vi "耐久性测试输出调用01.vi"(0 "电流":dbl, 5 "时长":dbl, 9 "字符串":string, 11 "输出簇":cluster{"电压1":refnum<vi>, "电流1":refnum<vi>}) -> ()   [LabVIEW 2020]
uses:
  <vilib>/Utility/miscctls.llb/LVDateTimeRec.ctl
panel:
  out "输出 3":dbl
  out "输出 2":dbl
  out "路径":path
  out "错误输出":errorcluster
  out "元素":string
  out "数值 3":i32
  out "Numeric":i32
  in  "数值":u32
  out "输出 1":dbl
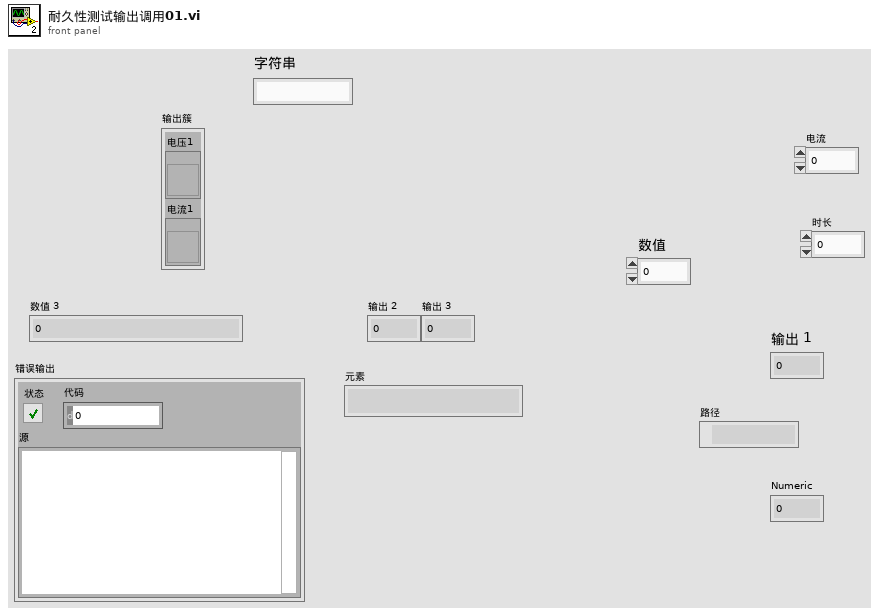
[diagram p1: front panel]
types:
  T1 = enum16{"open", "replace", "create", "open or create", "replace or create", "replace or create with confirmation"}
  T2 = typedef "LVDateTimeRec.ctl" = cluster{"fractional second":dbl, "second":i32, "minute":i32, "hour":i32, "day of month":i32, "month":i32, "year":i32, "day of week":i32, "day of year":i32, "DST":i32}
  T3 = enum16{"open", "open or create", "create or replace", "create", "open (read-only)"}
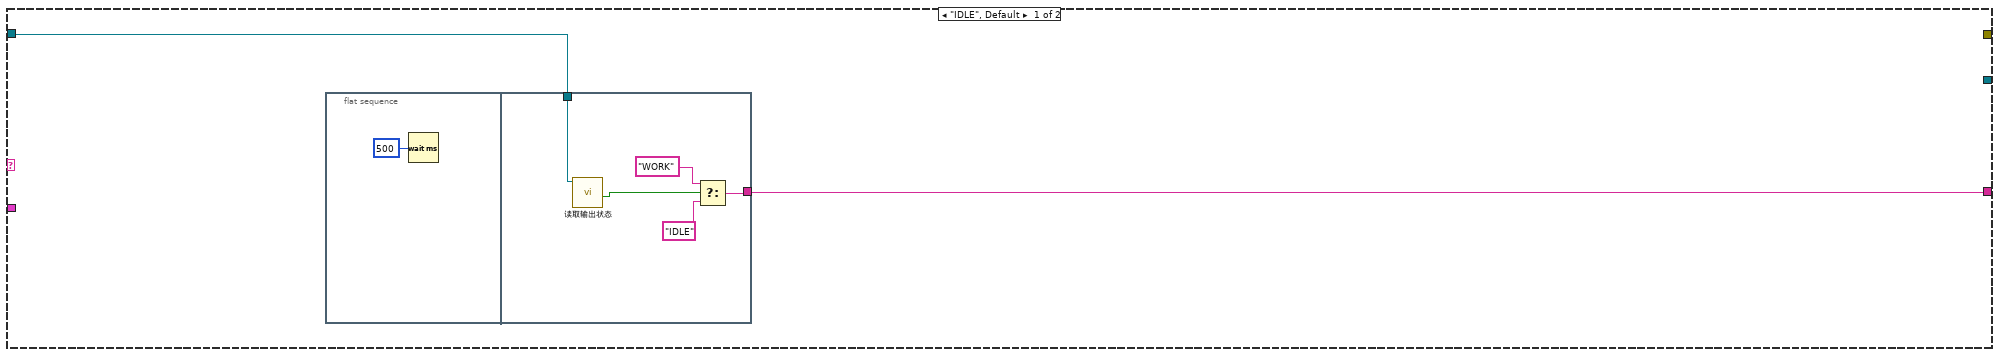
[diagram p2: hidden frame]
diagram:
  n1 = Current VI's Path() -> (path=w5:path)
  n2 = Strip Path(path=w5) -> (stripped path=w6:path)  [unwired: 1 out]
  n3 = Strip Path(path=w6) -> (stripped path=w7:path)  [unwired: 1 out]
  n4 = Path To String(path=w7) -> (string=w8:string)
  n5 = flat-sequence {
    tunnel: ["字符串"] -> w26
    tunnel: [w36] -> w27
    tunnel: w26 -> [w36]
    tunnel: [w44] -> w33
    tunnel: [w43] -> w32
    tunnel: [w42] -> w28
    tunnel: w27 -> [w41]
    tunnel: w33 -> [w54]
    tunnel: w32 -> [w53]
    tunnel: [w46] -> w31
    tunnel: [w45] -> w30
    tunnel: w31 -> [w93]
    tunnel: w30 -> [w92]
    tunnel: [w91] -> w29
    tunnel: [w90] -> w20
    tunnel: w29 -> [w121]
    tunnel: w20 -> [w119]
    frame #0 {
      n6 = property on="数值" class="DigNum (严格)"("Value"=i64 0 ("数值")) -> ()  [unwired: 2 in, 2 out]
    }
    frame #1 {
      n7 = VISA Close(VISA resource name="字符串") -> ()  [unwired: 1 in, 1 out]
    }
    frame #2 {
    }
    frame #3 {
      n8 = VISA Open(VISA resource name=w41) -> (VISA resource name=w42:refnum<visa-resource-name>, error out=w39:errorcluster)  [unwired: 4 in]
      n9 = call "remote.vi"("error in (no error)"=w39, "VISA resource name"=w42) -> ("error out"=w37:errorcluster, "VISA resource name out"=w38:refnum<visa-resource-name>)  [unwired: 8 in]
      n10 = call "enableoutput.vi"("error in (no error)"=w37, "Enable OutPut(True)"=FALSE, "VISA resource name"=w38) -> ("error out"=w43:errorcluster, "VISA resource name out"=w44:refnum<visa-resource-name>)  [unwired: 7 in]
    }
    frame #4 {
      n11 = flat-sequence {
        tunnel: w54 -> [w59]
        tunnel: w53 -> [w58]
        tunnel: [w56] -> w52
        tunnel: [w55] -> w51
        tunnel: w52 -> [w65]
        tunnel: w51 -> [w64]
        tunnel: [w61] -> w50
        tunnel: [w60] -> w49
        tunnel: w50 -> [w71]
        tunnel: w49 -> [w70]
        tunnel: [w68] -> w48
        tunnel: [w67] -> w47
        tunnel: w48 -> [w77]
        tunnel: w47 -> [w76]
        tunnel: [w73] -> w46
        tunnel: [w72] -> w45
        frame #0 {
          n12 = call "priority.vi"("error in (no error)"=w58, "字符串"="CURR", "VISA resource name"=w59) -> ("error out"=w55:errorcluster, "VISA resource name out"=w56:refnum<visa-resource-name>)  [unwired: 7 in]
        }
        frame #1 {
          n13 = call "初始化电压电流.vi"("error in (no error)"=w64, "输入 2"=0.1, "输入 1"=15.0, "VISA resource name"=w65) -> ("error out"=w60:errorcluster, "VISA resource name out"=w61:refnum<visa-resource-name>)  [unwired: 6 in]
        }
        frame #2 {
          n14 = call "限制电流.vi"("error in (no error)"=w70, "OCP Delay(0)"=3.0, "数值"=120.0 ("OCP Level(0)"), "VISA resource name"=w71) -> ("error out"=w67:errorcluster, "VISA resource name out"=w68:refnum<visa-resource-name>)  [unwired: 6 in]
        }
        frame #3 {
          n15 = call "限制电压.vi"("error in (no error)"=w76, "OVP Delay(0)"=3.0, "OVP Level(0)"=20.0, "VISA resource name"=w77) -> ("error out"=w72:errorcluster, "VISA resource name out"=w73:refnum<visa-resource-name>)  [unwired: 6 in]
        }
      }
    }
    frame #5 {
      n16 = flat-sequence {
        tunnel: w93 -> [w98]
        tunnel: w92 -> [w97]
        tunnel: [w96] -> w89
        tunnel: [w95] -> w88
        tunnel: "电流" -> [w94]
        tunnel: w89 -> [w101]
        tunnel: w88 -> [w102]
        tunnel: [w100] -> w87
        tunnel: [w99] -> w86
        tunnel: w80 -> [w112]
        tunnel: w87 -> [w111]
        tunnel: [w111] -> w85
        tunnel: [w110] -> w84
        tunnel: w86 -> [w110]
        tunnel: w85 -> [w114]
        tunnel: [w114] -> w83
        tunnel: w84 -> [w113]
        tunnel: [w113] -> w82
        tunnel: [w117] -> w91
        tunnel: w83 -> [w118]
        tunnel: w82 -> [w116]
        tunnel: [w115] -> w90
        frame #0 {
          n17 = call "设置电流.vi"("error in (no error)"=w97, "输入 1"=w94, "VISA resource name"=w98) -> ("error out"=w95:errorcluster, "VISA resource name out"=w96:refnum<visa-resource-name>)  [unwired: 7 in]
        }
        frame #1 {
          n18 = First Call?() -> (First Call?: T/F=w103:bool)
          n19 = case shown="真" w103 {
            tunnel: w101 -> [w104 w109]
            tunnel: w102 -> [_ w108]
            tunnel: [w104 w106] -> w100
            tunnel: [_ w105] -> w99
            frame False {
            }
            frame True {
              n20 = call "enableoutput.vi"("error in (no error)"=w108, "Enable OutPut(True)"=TRUE, "VISA resource name"=w109) -> ("error out"=w105:errorcluster, "VISA resource name out"=w106:refnum<visa-resource-name>)  [unwired: 7 in]
            }
          }
        }
        frame #2 {
          n21 = Wait (ms)(milliseconds to wait=w112) -> ()  [unwired: 1 out]
        }
        frame #3 {
        }
        frame #4 {
          n22 = call "remote.vi"("error in (no error)"=w116, "VISA resource name"=w118) -> ("error out"=w115:errorcluster, "VISA resource name out"=w117:refnum<visa-resource-name>)  [unwired: 8 in]
        }
      }
      n23 = Multiply(x="时长", y=3600000.0) -> (x*y=w80:dbl)
      "输出 1" <- "电流"
    }
    frame #6 {
      n24 = flat-sequence {
        tunnel: w121 -> [w125]
        tunnel: [w124] -> w120
        tunnel: w119 -> [w122]
        tunnel: w120 -> [w126]
        frame #0 {
          n25 = call "enableoutput.vi"("error in (no error)"=w122, "Enable OutPut(True)"=FALSE, "VISA resource name"=w125) -> ("VISA resource name out"=w124:refnum<visa-resource-name>)  [unwired: 7 in, 1 out]
        }
        frame #1 {
          n26 = VISA Close(VISA resource name=w126) -> ()  [unwired: 1 in, 1 out]
        }
        frame #2 {
          n27 = flat-sequence {
            tunnel: [w140] -> w132
            tunnel: [w139] -> w131
            tunnel: [w138] -> w130
            tunnel: w132 -> [w164]
            tunnel: w131 -> [w165]
            tunnel: [w164] -> w127
            tunnel: [w165] -> w128
            tunnel: w130 -> [w163]
            tunnel: [w163] -> w129
            tunnel: w129 -> [w188]
            tunnel: w128 -> [w192]
            tunnel: w127 -> [w191]
            frame #0 {
              n28 = property on="路径" class="Path"() -> ("Value"=w137:path)  [unwired: 2 in, 2 out]
              n29 = Open/Create/Replace File(file path (use dialog)=w137, operation (0:open)=T1."open" ("操作(0:open)")) -> (refnum out=w142:refnum<file>, error out=w141:errorcluster)  [unwired: 4 in, 1 out]
              n30 = Read from Text File(file (use dialog)=w142, count=-1 ("计数"), error in=w141) -> (refnum out=w135:refnum<file>, text=w136:string[], error out=w133:errorcluster)  [unwired: 1 in, 1 out]
              n31 = for {
                tunnel: [w148] -> w140 mode=indexing
                tunnel: [w147] -> w139 mode=indexing
                tunnel: [w151] -> w138 mode=indexing
                tunnel: w136 -> [w144] mode=indexing
                i -> [w146]
                n32 = Search/Split String(string=w144, search string/char (-)="电流：" ("正则表达式")) -> (substring before match=w159:string, match + rest of string=w150:string)  [unwired: 1 in, 1 out]
                n33 = Scan From String(format string="%d-%d-%d %d:%d:%d" ("格式字符串"), input string=w159) -> (output 1=w158:i32, output 2=w157:i32, output 3=w156:i32, output 4=w155:i32, output 5=w154:i32, output 6=w153:i32)  [unwired: 8 in, 3 out]
                n34 = Bundle By Name(cluster=T2 {"fractional second"=0.9035696983337402, "second"=34, "minute"=35, "hour"=15, "day of month"=21, "month"=2, "year"=2022, "day of week"=2, "day of year"=52, "DST"=0} ("日期时间记录"), "second"=w153, "minute"=w154, "hour"=w155, "day of month"=w156, "month"=w157, "year"=w158) -> (w152:T2)
                n35 = Scan From String(format string="电流：%f 电压：%f" ("格式字符串"), input string=w150) -> (error out=w145:errorcluster, output 1=w148:dbl, output 2=w147:dbl)  [unwired: 4 in, 2 out]
                n36 = call <vilib>:"Clear Errors.vi"("error in (no error)"=w145) -> ()  [unwired: 5 in, 2 out]
                n37 = Date/Time To Seconds(2:w152) -> (0:w151:timestamp)  [unwired: 1 in]
                "元素" <- w144
                "数值 3" <- w146
              }
              n38 = Close File(refnum=w135, error in=w133) -> ()  [unwired: 2 out]
            }
            frame #1 {
            }
            frame #2 {
              w182 = "数据" ("组名称")
              n39 = Array Size(array=w188) -> (size(s)=w187:i32)
              n40 = Array Max & Min(array=w192) -> (max value=w205:dbl, max index (indices)=w200:i32, min value=w204:dbl, min index (indices)=w199:i32)
              n41 = Array Max & Min(array=w191) -> (max value=w207:dbl, max index (indices)=w201:i32, min value=w208:dbl, min index (indices)=w202:i32)
              n42 = Index Array(array=w188, index=0 ("索引")) -> (element=w185:timestamp)
              n43 = Decrement(x=w187) -> (x-1=w186:i32)
              n44 = Build Array(w204, w205, w200, w199) -> (w203:dbl[])
              n45 = Build Array(w208, w207, w202, w201) -> (w206:dbl[])
              n46 = Index Array(array=w188, index=w186) -> (element=w184:timestamp)
              n47 = call <vilib>:"Application Directory.vi"() -> ("Application Directory"=w166:path)
              n48 = Path To String(path=w166) -> (string=w171:string)
              n49 = Get Date/Time In Seconds() -> (seconds since 1Jan1904=w224:timestamp)
              n50 = Format Date/Time String(time format string (%c)="%Y-%m-%d-%H-%M-%S" ("时间格式字符串(%c)"), seconds (now)=w224) -> (date/time string=w173:string)  [unwired: 1 in]
              n51 = Concatenate Strings(w171, "\\" ("字符串"), w173, ".tdms" ("字符串")) -> (w225:string)
              n52 = String To Path(string=w225) -> (path=w226:path)
              n53 = Build Array(w185, w184) -> (w183:timestamp[])
              n54 = TDMS Open(5:FALSE ("创建索引文件？(T)"), 10:T3."create or replace" ("操作(0:open)"), 11:w226) -> (0:w179:errorcluster, 3:w181:refnum<k34>)  [unwired: 4 in]
              n55 = Build Array("电解水实验" ("组名称"), "孙成，王彪" ("组名称"), w173, "极化曲线" ("组名称")) -> (w172:string[])
              n56 = TDMS Set Properties(5:w172, 7:string[] ["Title", "Author", "Date/Time", "type"] ("属性名称"), 8:w179, 11:w181) -> (0:w178:errorcluster, 3:w180:refnum<k34>)  [unwired: 2 in, 2 out]
              n57 = TDMS Set Properties(5:w183, 7:string[] ["最小值", "最大值"] ("属性名称"), 8:w178, 9:"测试时间" ("通道名称"), 10:w182, 11:w180) -> (0:w215:errorcluster, 3:w216:refnum<k34>)  [unwired: 2 out]
              n58 = TDMS Set Properties(5:w206, 7:string[] ["最小值", "最大值", "最小索引", "最大索引"] ("属性名称"), 8:w215, 9:"电流" ("通道名称"), 10:w182, 11:w216) -> (0:w209:errorcluster, 3:w212:refnum<k34>)  [unwired: 2 out]
              n59 = TDMS Set Properties(5:w203, 7:string[] ["最小值", "最大值", "最小索引", "最大索引"] ("属性名称"), 8:w209, 9:"电压" ("通道名称"), 10:w182, 11:w212) -> (0:w167:errorcluster, 3:w168:refnum<k34>)  [unwired: 2 out]
              n60 = TDMS Write(0:w168, 5:"数据" ("组名称输入（无标题）"), 7:string[] ["电流"] ("通道名输入（无标题）"), 9:w191, 11:w167) -> (4:w195:refnum<k34>, 15:w194:errorcluster)  [unwired: 1 in, 2 out]
              n61 = TDMS Write(0:w195, 5:"数据" ("组名称输入（无标题）"), 7:string[] ["电压"] ("通道名输入（无标题）"), 9:w192, 11:w194) -> (4:w170:refnum<k34>, 15:w169:errorcluster)  [unwired: 1 in, 2 out]
              n62 = TDMS Close(8:w169, 11:w170) -> (0:→"错误输出":errorcluster)  [unwired: 1 out]
            }
          }
        }
        frame #3 {
          n63 = Request Deallocation(TRUE ("标志")) -> ()
        }
        frame #4 {
          n64 = Stop(stop? (T)=TRUE ("停止？(T)")) -> ()
        }
      }
    }
  }
  n65 = Get Date/Time In Seconds() -> (seconds since 1Jan1904=w10:timestamp)
  n66 = Format Date/Time String(time format string (%c)="%y-%m-%d[%H-%M]", seconds (now)=w10) -> (date/time string=w13:string)  [unwired: 1 in]
  n67 = Concatenate Strings(w8, "\\" ("string"), "耐久性\\" ("string"), w13) -> (w3:string)
  n68 = String To Path(string=w3) -> (path=w4:path)
  n69 = Create Folder(path (use dialog)=w4) -> (created path=w2:path)  [unwired: 2 in, 2 out]
  n70 = Path To String(path=w2) -> (string=w17:string)
  n71 = Concatenate Strings(w17, "\\" ("string"), "数据.txt" ("string")) -> (w16:string)
  n72 = String To Path(string=w16) -> (path=w15:path)
  "路径" <- w15
  n73 = Open/Create/Replace File(file path (use dialog)=w15, operation (0:open)=T1."replace or create" ("操作(0:open)")) -> (refnum out=w14:refnum<file>, error out=w23:errorcluster)  [unwired: 4 in, 1 out]
  n74 = while {
    shift-right: [w232] -> _
    shift-left: "IDLE" -> [w238]
    tunnel: w28 -> [w237]
    tunnel: w14 -> [w236]
    tunnel: w23 -> [w235]
    tunnel: [w234] -> w22
    tunnel: [w233] -> w21
    tunnel: "输出簇" -> [w229]
    i -> [w231]
    stop <- FALSE stop-if-true
    n75 = Wait (ms)(milliseconds to wait=u32 500 ("等待时间（毫秒）")) -> ()  [unwired: 1 out]
    n76 = case shown="\"WORK\"" w238 {
      tunnel: [w241 w269] -> w232
      tunnel: w237 -> [w240 w277]
      tunnel: w236 -> [_ w276]
      tunnel: w235 -> [_ w274]
      tunnel: [_ w271] -> w234
      tunnel: [_ w270] -> w233
      tunnel: w229 -> [_ w250]
      frame "IDLE", Default {
        n77 = flat-sequence {
          tunnel: [w244] -> w241
          tunnel: w240 -> [w243]
          frame #0 {
            n78 = Wait (ms)(milliseconds to wait=u32 500 ("等待时间（毫秒）")) -> ()  [unwired: 1 out]
          }
          frame #1 {
            n79 = call "读取输出状态.vi"("VISA resource name"=w243) -> ("x = y?"=w247:bool)  [unwired: 7 in, 3 out]
            n80 = Select(t="WORK", s=w247, f="IDLE") -> (s? t:f=w244:string)
          }
        }
      }
      frame "WORK" {
        n81 = Unbundle By Name(w250) -> ("电压1"=w248:refnum<vi>, "电流1"=w249:refnum<vi>)
        n82 = flat-sequence {
          tunnel: [w286] -> w280
          tunnel: [w285] -> w279
          tunnel: w277 -> [w284]
          tunnel: w276 -> [w282]
          tunnel: [w283] -> w275
          tunnel: w274 -> [w283]
          tunnel: [w282] -> w273
          tunnel: [w281] -> w272
          tunnel: w280 -> [w298]
          tunnel: w279 -> [w297]
          tunnel: [w295] -> w268
          tunnel: [w294] -> w266
          tunnel: w275 -> [w292]
          tunnel: w273 -> [w293]
          tunnel: [w293] -> w264
          tunnel: [w292] -> w262
          tunnel: [w288] -> w260
          tunnel: w272 -> [_]
          tunnel: [w288] -> w258
          tunnel: w268 -> [w312]
          tunnel: [w312] -> w267
          tunnel: w266 -> [w311]
          tunnel: [w311] -> w265
          tunnel: w264 -> [w310]
          tunnel: [w310] -> w263
          tunnel: w262 -> [w309]
          tunnel: [w309] -> w261
          tunnel: w260 -> [w306]
          tunnel: [w306] -> w259
          tunnel: w258 -> [w301]
          tunnel: [w301] -> w257
          tunnel: w249 -> [w308]
          tunnel: w248 -> [w304]
          tunnel: [w338] -> w256
          tunnel: w267 -> [w338]
          tunnel: w265 -> [w321]
          tunnel: w263 -> [w325]
          tunnel: w261 -> [w324]
          tunnel: w259 -> [w323]
          tunnel: w257 -> [w319]
          tunnel: [w322] -> w254
          tunnel: [w321] -> w252
          tunnel: [w320] -> w270
          tunnel: w256 -> [w341]
          tunnel: [w341] -> w255
          tunnel: w254 -> [w340]
          tunnel: [w340] -> w253
          tunnel: w252 -> [w339]
          tunnel: [w339] -> w251
          tunnel: [w345] -> w278
          tunnel: w255 -> [w345]
          tunnel: w253 -> [w344]
          tunnel: w251 -> [w343]
          tunnel: [w342] -> w271
          tunnel: w278 -> [w350]
          tunnel: [w346] -> w269
          frame #0 {
            w287 = 0 items=["Current", "Power", "Voltage", "Capacity", "Temperature", "Time"] ("Fetch Type")
            n83 = call "fetch.vi"("Fetch Type"=w287, "VISA resource name"=w284) -> ("error out"=w285:errorcluster, "输出 1"=w281:dbl, "VISA resource name out"=w286:refnum<visa-resource-name>)  [unwired: 7 in]
            "输出 2" <- w281
          }
          frame #1 {
            w296 = 2 items=["Current", "Power", "Voltage", "Capacity", "Temperature", "Time"] ("Fetch Type")
            n84 = Random Number (0-1)() -> (number: 0 to 1=w290:dbl)
            n85 = call "fetch.vi"("error in (no error)"=w297, "Fetch Type"=w296, "VISA resource name"=w298) -> ("error out"=w294:errorcluster, "输出 1"=→"输出 3":dbl, "VISA resource name out"=w295:refnum<visa-resource-name>)  [unwired: 6 in]
            n86 = Multiply(x=w290, y=10.0) -> (x*y=w288:dbl)
          }
          frame #2 {
            n87 = property class="Arr (严格)"(reference=w308) -> (reference out=w300:refnum<vi>, "Value"=w307:dbl[])  [unwired: 1 in, 1 out]
            n88 = property class="Arr (严格)"(reference=w304) -> (reference out=w299:refnum<vi>, "Value"=w303:dbl[])  [unwired: 1 in, 1 out]
            n89 = Insert Into Array(array=w303, new element=w301) -> (w302:dbl[])  [unwired: 1 in]
            n90 = Insert Into Array(array=w307, new element=w306) -> (w305:dbl[])  [unwired: 1 in]
            n91 = property class="Arr (严格)"(reference=w299, "Value"=w302) -> ()  [unwired: 1 in, 2 out]
            n92 = property class="Arr (严格)"(reference=w300, "Value"=w305) -> ()  [unwired: 1 in, 2 out]
          }
          frame #3 {
            n93 = Format Into String(w323) -> (resulting string=w334:string)  [unwired: 3 in, 1 out]
            n94 = Get Date/Time In Seconds() -> (seconds since 1Jan1904=w337:timestamp)
            n95 = Format Date/Time String(time format string (%c)="%Y-%m-%d %H:%M:%S" ("时间格式字符串(%c)"), seconds (now)=w337) -> (date/time string=w335:string)  [unwired: 1 in]
            n96 = Format Into String(w319) -> (resulting string=w329:string)  [unwired: 3 in, 1 out]
            n97 = call <vilib>:"Space Constant.vi"() -> ("String"=w318:string)
            n98 = Write to Text File(file (use dialog)=w325, text=w335, error in=w324) -> (refnum out=w332:refnum<file>, error out=w331:errorcluster)  [unwired: 1 in, 1 out]
            n99 = Concatenate Strings(w318, "电流：" ("字符串"), w334) -> (w333:string)
            n100 = call <vilib>:"Space Constant.vi"() -> ("String"=w317:string)
            n101 = Write to Text File(file (use dialog)=w332, text=w333, error in=w331) -> (refnum out=w328:refnum<file>, error out=w327:errorcluster)  [unwired: 1 in, 1 out]
            n102 = Concatenate Strings(w317, "电压：" ("字符串"), w329) -> (w330:string)
            n103 = Write to Text File(file (use dialog)=w328, text=w330, error in=w327) -> (refnum out=w314:refnum<file>, error out=w313:errorcluster)  [unwired: 1 in, 1 out]
            n104 = Write to Text File(file (use dialog)=w314, text="\r\n", error in=w313) -> (refnum out=w320:refnum<file>, error out=w322:errorcluster)  [unwired: 1 in, 1 out]
          }
          frame #4 {
          }
          frame #5 {
            n105 = Merge Errors(w343, w344) -> (w342:errorcluster)
          }
          frame #6 {
            n106 = call "读取输出状态.vi"("VISA resource name"=w350) -> ("x = y?"=w349:bool)  [unwired: 7 in, 3 out]
            n107 = Select(t="WORK", s=w349, f="IDLE") -> (s? t:f=w346:string)
          }
        }
      }
    }
    "Numeric" <- w231
  }
  n108 = Close File(refnum=w21, error in=w22) -> ()  [unwired: 2 out]
